vi "num50-150.vi"() -> ()   [LabVIEW 2013]
panel:
  out "Contador":dbl
  out "Numero 50-150":dbl
  # "Generar 10 numeros entre 50-150 , usar un ciclo while\npara validar que el numero se encuentre en ese rango \nantes de presentarlos.\nIr contando los numeros."
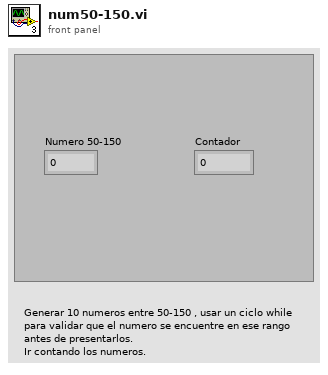
[diagram p1: front panel]
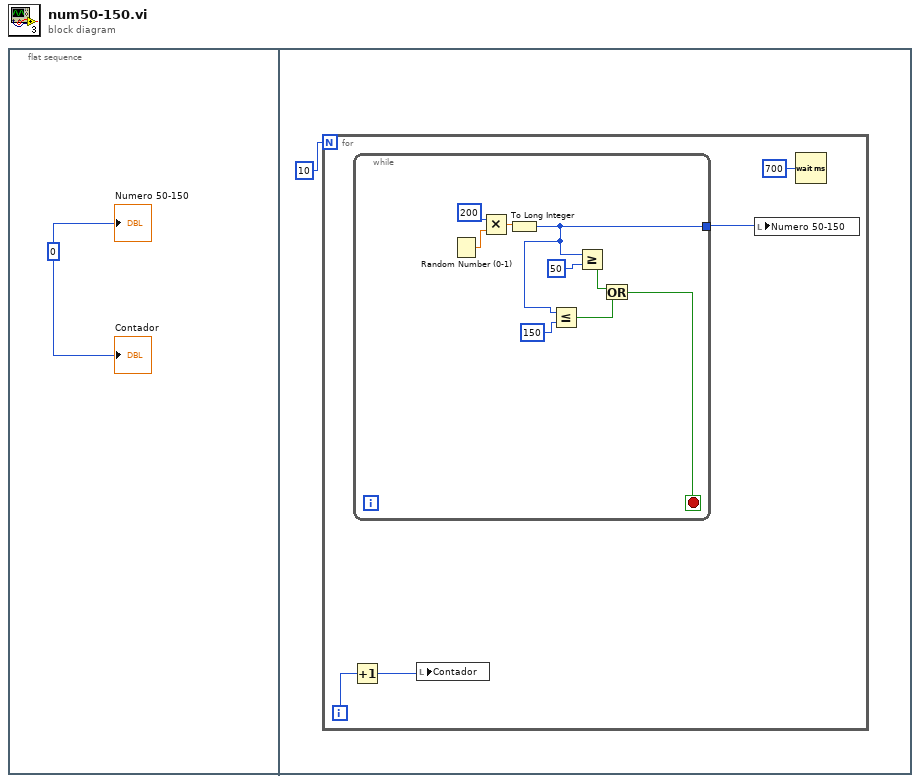
[diagram p0: block diagram]
diagram:
  n1 = flat-sequence {
    frame #0 {
      w1 = 0
      "Numero 50-150" <- w1
      "Contador" <- w1
    }
    frame #1 {
      n2 = for {
        N: 10 -> [_]
        i -> [w5]
        n3 = Increment(x=w5) -> (x+1=w4:i32)
        n4 = while {
          tunnel: [w11] -> w6
          stop <- w7 stop-if-true
          n5 = Random Number (0-1)() -> (number: 0 to 1=w14:dbl)
          n6 = Multiply(x=200, y=w14) -> (x*y=w13:dbl)
          n7 = To Long Integer(number=w13) -> (32bit integer=w11:i32)
          n8 = Less Or Equal?(x=w11, y=150) -> (x <= y?=w8:bool)
          n9 = Greater Or Equal?(x=w11, y=50) -> (x >= y?=w9:bool)
          n10 = Or(x=w9, y=w8) -> (x .or. y?=w7:bool)
        }
        n11 = local write "Contador"(w4) -> ()
        n12 = local write "Numero 50-150"(w6) -> ()
        n13 = Wait (ms)(milliseconds to wait=u32 700) -> ()  [unwired: 1 out]
      }
    }
  }
